vi "Set Source Property Count.vi"(7 "Source Index":i32, 8 "error in (no error)":errorcluster, 10 "Properties Count":i32, 11 "BuildSpec in":refnum<vi>) -> (0 "error out":errorcluster, 3 "BuildSpec out":refnum<vi>)   [LabVIEW 2019, in "Project Sync Tools.lvclass"]
uses:
  Project Sync Tools.lvclass
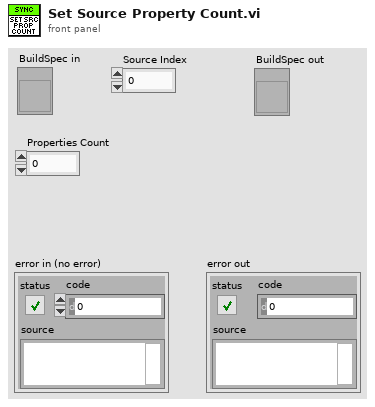
[diagram p1: front panel]
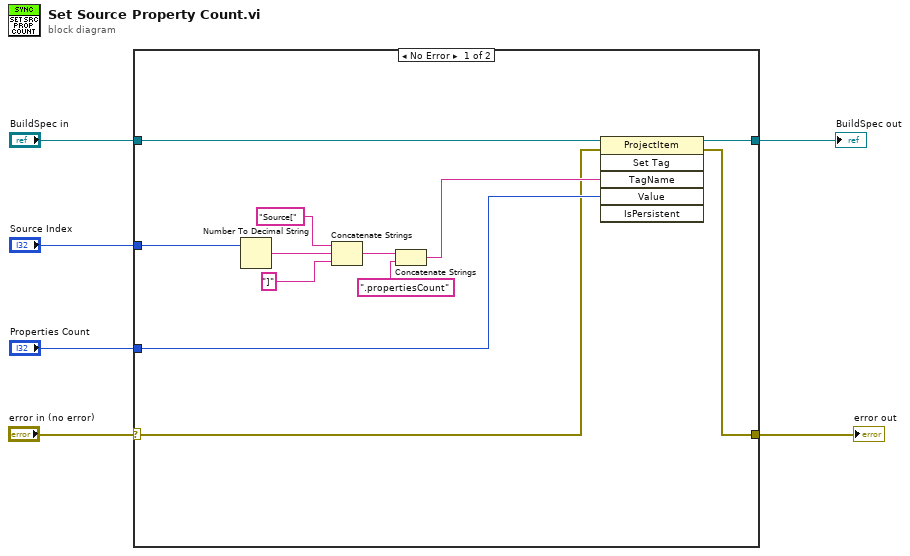
[diagram p0: block diagram]
diagram:
  n1 = case shown="No Error" "error in (no error)" {
    selector: "error in (no error)" -> [w7 w20]
    tunnel: "Properties Count" -> [w18 _]
    tunnel: "Source Index" -> [w16 _]
    tunnel: [w10 w19] -> w4
    tunnel: "BuildSpec in" -> [w9 w19]
    tunnel: [w8 w20] -> w2
    frame No Error {
      n2 = Number To Decimal String(number=w16) -> (decimal integer string=w13:string)  [unwired: 1 in]
      n3 = Concatenate Strings("Source[" ("string"), w13, "]") -> (w15:string)
      n4 = Concatenate Strings(w15, ".propertiesCount") -> (w17:string)
      n5 = invoke class="ProjectItem" method="Set Tag"(reference=w9, error in=w7, "TagName"=w17, "Value"=w18) -> (reference out=w10:refnum<vi>, error out=w8:errorcluster)  [unwired: 2 in, 4 out]
    }
    frame Error {
    }
  }
  "BuildSpec out" <- w4
  "error out" <- w2
